vi "Pane Relief Main UI.vi"(8 "Error In":errorcluster, 10 "Stopped Event":refnum<user-event>, 11 "QD Launch VI Ref":refnum<vi>) -> (0 "Error Out":errorcluster, 3 "Pane Relief Main UI out":refnum<class "Pane Relief Main UI.lvclass">)   [LabVIEW 2018, in "Pane Relief Main UI.lvlib" / "Pane Relief Main UI.lvclass"]
uses:
  <resource>/dialog/QuickDrop/plugins/PaneRelief/Classes/Pane Relief Main UI/Pane Relief Main UI/Pane Relief Main UI.lvclass
  <resource>/dialog/QuickDrop/plugins/PaneRelief/Classes/Pane Relief Main UI/Pane Relief Main UI/Pane Relief Main UI.lvclass/Pane Relief Main UI.ctl
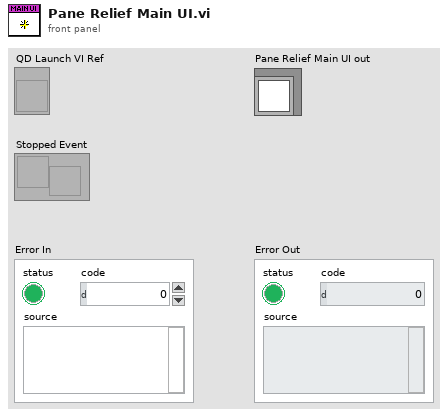
[diagram p1: front panel]
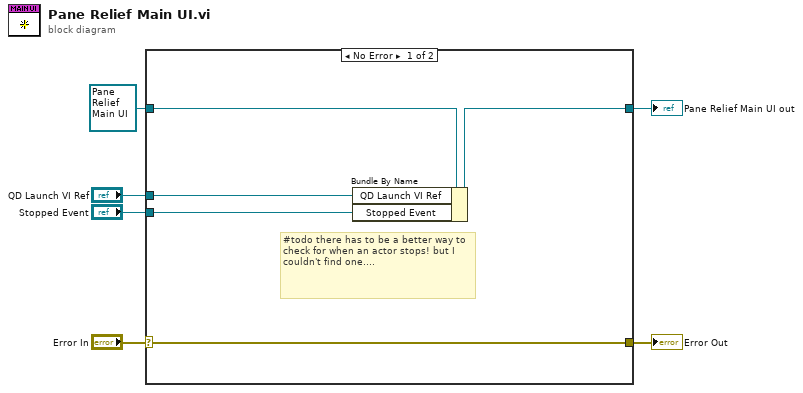
[diagram p0: block diagram]
diagram:
  n1 = case shown="No Error" "Error In" {
    selector: "Error In" -> [w11 w13]
    tunnel: [w11 w13] -> w4
    tunnel: [w10 w12] -> w6
    tunnel: refnum<class "Pane Relief Main UI.lvclass"> refnum ("Pane Relief Main UI in") -> [w9 w12]
    tunnel: "QD Launch VI Ref" -> [w8 _]
    tunnel: "Stopped Event" -> [w7 _]
    frame No Error {
      # "#todo there has to be a better way to check for when an actor stops! but I couldn't find one...."
      n2 = Bundle By Name(cluster=w9, "QD Launch VI Ref"=w8, "Stopped Event"=w7) -> (w10:refnum<class "Pane Relief Main UI.lvclass">)
    }
    frame Error {
    }
  }
  "Pane Relief Main UI out" <- w6
  "Error Out" <- w4
